vi "GUI.VISAResourceName.Set.vi"(8 "error in (no error)":errorcluster, 10 "deviceVISAConnect":refnum<visa-resource-name>, 11 "deviceVISAName":string) -> (0 "error out":errorcluster)   [LabVIEW 2019]
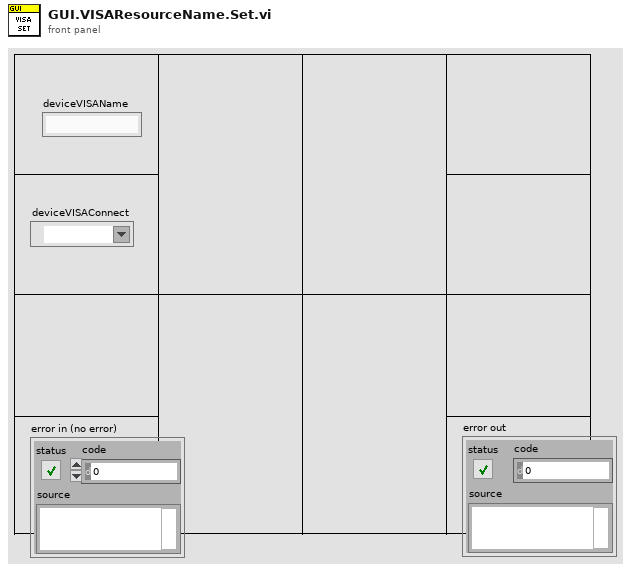
[diagram p1: front panel]
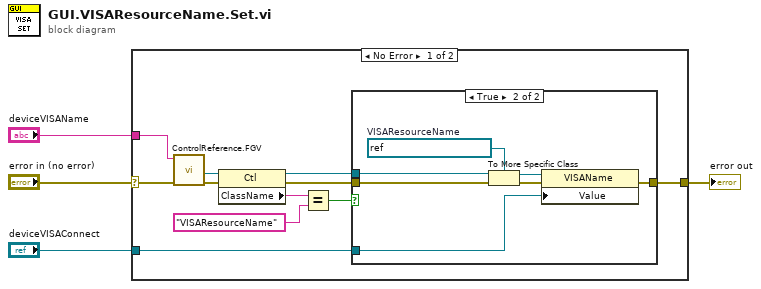
[diagram p0: block diagram]
diagram:
  n1 = case shown="No Error" "error in (no error)" {
    selector: "error in (no error)" -> [w9 w24]
    tunnel: [w10 w24] -> w2
    tunnel: "deviceVISAName" -> [w7 _]
    tunnel: "deviceVISAConnect" -> [w11 _]
    frame No Error {
      n2 = call "ControlReference.FGV.vi"("error in (no error)"=w9, "controlLabelText"=w7) -> ("error out"=w8:errorcluster, "referenceToControl"=w6:refnum<vi>)  [unwired: 8 in]
      n3 = property class="Ctl"(reference=w6, error in=w8) -> (reference out=w13:refnum<vi>, error out=w12:errorcluster, "ClassName"=w5:string)
      n4 = Equal?(x=w5, y="VISAResourceName") -> (x = y?=w14:bool)
      n5 = case shown="True" w14 {
        tunnel: w13 -> [_ w22]
        tunnel: w12 -> [w16 w23]
        tunnel: w11 -> [_ w18]
        tunnel: [w16 w17] -> w10
        frame False {
        }
        frame True {
          w21 = refnum<vi> refnum  # VISAResourceName
          n6 = To More Specific Class(target class=w21, reference=w22, error in=w23) -> (specific class reference=w20:refnum<vi>, error out=w19:errorcluster)
          n7 = property class="VISAName"(reference=w20, error in=w19, "Value"=w18) -> (error out=w17:errorcluster)  [unwired: 1 out]
        }
      }
    }
    frame Error {
    }
  }
  "error out" <- w2
